vi "Test - Draw Teapot.vi"() -> ()   [LabVIEW 2022 SP3, in "Raster.lvlib"] (continued)
"v"=0.0}, "Colour"=12517256}, "Vertex 3"={"Position"={"x"=400.0, "y"=464.85934, "z"=0.98939073}, "UV"={"u"=0.0, "v"=0.0}, "Colour"=12517256}, "Alpha"=0.0, "Alpha Blending Enabled"=FALSE, "Colour"=12385414}, {"Vertex 1"={"Position"={"x"=261.91296, "y"=120.87895, "z"=0.98915625}, "UV"={"u"=0.0, "v"=0.0}, "Colour"=12517256}, "Vertex 2"={"Position"={"x"=278.23944, "y"=120.85737, "z"=0.98926175}, "UV"={"u"=0.0, "v"=0.0}, "Colour"=12517256}, "Vertex 3"={"Position"={"x"=278.11005, "y"=127.45417, "z"=0.9896591}, "UV"={"u"=0.0, "v"=0.0}, "Colour"=12517256}, "Alpha"=0.0, "Alpha Blending Enabled"=FALSE, "Colour"=131841}, {"Vertex 1"={"Position"={"x"=411.51666, "y"=449.75494, "z"=0.98939085}, "UV"={"u"=0.0, "v"=0.0}, "Colour"=12517256}, "Vertex 2"={"Position"={"x"=412.7883, "y"=456.74655, "z"=0.98931825}, "UV"={"u"=0.0, "v"=0.0}, "Colour"=12517256}, "Vertex 3"={"Position"={"x"=418.46112, "y"=456.03012, "z"=0.9893673}, "UV"={"u"=0.0, "v"=0.0}, "Colour"=12517256}, "Alpha"=0.0, "Alpha Blending Enabled"=FALSE, "Colour"=2240024}, {"Vertex 1"={"Position"={"x"=561.44336, "y"=135.88576, "z"=0.9895325}, "UV"={"u"=0.0, "v"=0.0}, "Colour"=12517256}, "Vertex 2"={"Position"={"x"=559.66595, "y"=133.57411, "z"=0.9895382}, "UV"={"u"=0.0, "v"=0.0}, "Colour"=12517256}, "Vertex 3"={"Position"={"x"=561.4089, "y"=125.13941, "z"=0.98900545}, "UV"={"u"=0.0, "v"=0.0}, "Colour"=12517256}, "Alpha"=0.0, "Alpha Blending Enabled"=FALSE, "Colour"=131841}, {"Vertex 1"={"Position"={"x"=358.07327, "y"=408.73547, "z"=0.9892421}, "UV"={"u"=0.0, "v"=0.0}, "Colour"=12517256}, "Vertex 2"={"Position"={"x"=369.4374, "y"=409.63797, "z"=0.98946077}, "UV"={"u"=0.0, "v"=0.0}, "Colour"=12517256}, "Vertex 3"={"Position"={"x"=374.2221, "y"=410.54718, "z"=0.98937297}, "UV"={"u"=0.0, "v"=0.0}, "Colour"=12517256}, "Alpha"=0.0, "Alpha Blending Enabled"=FALSE, "Colour"=10014061}, {"Vertex 1"={"Position"={"x"=238.15663, "y"=384.24957, "z"=0.9895312}, "UV"={"u"=0.0, "v"=0.0}, "Colour"=12517256}, "Vertex 2"={"Position"={"x"=240.3879, "y"=388.06317, "z"=0.98953843}, "UV"={"u"=0.0, "v"=0.0}, "Colour"=12517256}, "Vertex 3"={"Position"={"x"=238.64832, "y"=392.52478, "z"=0.9890058}, "UV"={"u"=0.0, "v"=0.0}, "Colour"=12517256}, "Alpha"=0.0, "Alpha Blending Enabled"=FALSE, "Colour"=6126658}, {"Vertex 1"={"Position"={"x"=414.14594, "y"=412.64026, "z"=0.98952574}, "UV"={"u"=0.0, "v"=0.0}, "Colour"=12517256}, "Vertex 2"={"Position"={"x"=420.22992, "y"=411.29608, "z"=0.9893006}, "UV"={"u"=0.0, "v"=0.0}, "Colour"=12517256}, "Vertex 3"={"Position"={"x"=414.01163, "y"=411.85974, "z"=0.9892462}, "UV"={"u"=0.0, "v"=0.0}, "Colour"=12517256}, "Alpha"=0.0, "Alpha Blending Enabled"=FALSE, "Colour"=10804598}, {"Vertex 1"={"Position"={"x"=412.7883, "y"=456.74655, "z"=0.98931825}, "UV"={"u"=0.0, "v"=0.0}, "Colour"=12517256}, "Vertex 2"={"Position"={"x"=411.51666, "y"=449.75494, "z"=0.98939085}, "UV"={"u"=0.0, "v"=0.0}, "Colour"=12517256}, "Vertex 3"={"Position"={"x"=405.94202, "y"=450.1419, "z"=0.98936325}, "UV"={"u"=0.0, "v"=0.0}, "Colour"=12517256}, "Alpha"=0.0, "Alpha Blending Enabled"=FALSE, "Colour"=2635293}, {"Vertex 1"={"Position"={"x"=400.0, "y"=462.5336, "z"=0.98927724}, "UV"={"u"=0.0, "v"=0.0}, "Colour"=12517256}, "Vertex 2"={"Position"={"x"=400.0, "y"=464.85934, "z"=0.98939073}, "UV"={"u"=0.0, "v"=0.0}, "Colour"=12517256}, "Vertex 3"={"Position"={"x"=405.62814, "y"=464.7204, "z"=0.9893997}, "UV"={"u"=0.0, "v"=0.0}, "Colour"=12517256}, "Alpha"=0.0, "Alpha Blending Enabled"=FALSE, "Colour"=12385414}, {"Vertex 1"={"Position"={"x"=240.33403, "y"=133.57411, "z"=0.9895382}, "UV"={"u"=0.0, "v"=0.0}, "Colour"=12517256}, "Vertex 2"={"Position"={"x"=238.55664, "y"=135.88576, "z"=0.9895325}, "UV"={"u"=0.0, "v"=0.0}, "Colour"=12517256}, "Vertex 3"={"Position"={"x"=236.70218, "y"=127.47084, "z"=0.9889933}, "UV"={"u"=0.0, "v"=0.0}, "Colour"=12517256}, "Alpha"=0.0, "Alpha Blending Enabled"=FALSE, "Colour"=131841}, {"Vertex 1"={"Position"={"x"=327.3322, "y"=123.64719, "z"=0.9895792}, "UV"={"u"=0.0, "v"=0.0}, "Colour"=12517256}, "Vertex 2"={"Position"={"x"=299.91116, "y"=121.74838, "z"=0.98940194}, "UV"={"u"=0.0, "v"=0.0}, "Colour"=12517256}, "Vertex 3"={"Position"={"x"=303.40628, "y"=116.389046, "z"=0.98908174}, "UV"={"u"=0.0, "v"=0.0}, "Colour"=12517256}, "Alpha"=0.0, "Alpha Blending Enabled"=FALSE, "Colour"=131841}, {"Vertex 1"={"Position"={"x"=559.61206, "y"=388.06317, "z"=0.98953843}, "UV"={"u"=0.0, "v"=0.0}, "Colour"=12517256}, "Vertex 2"={"Position"={"x"=561.8434, "y"=384.24957, "z"=0.9895312}, "UV"={"u"=0.0, "v"=0.0}, "Colour"=12517256}, "Vertex 3"={"Position"={"x"=563.7232, "y"=388.5807, "z"=0.9889904}, "UV"={"u"=0.0, "v"=0.0}, "Colour"=12517256}, "Alpha"=0.0, "Alpha Blending Enabled"=FALSE, "Colour"=6126658}, {"Vertex 1"={"Position"={"x"=561.8434, "y"=138.31693, "z"=0.9895312}, "UV"={"u"=0.0, "v"=0.0}, "Colour"=12517256}, "Vertex 2"={"Position"={"x"=561.44336, "y"=135.88576, "z"=0.9895325}, "UV"={"u"=0.0, "v"=0.0}, "Colour"=12517256}, "Vertex 3"={"Position"={"x"=563.29785, "y"=127.47084, "z"=0.9889933}, "UV"={"u"=0.0, "v"=0.0}, "Colour"=12517256}, "Alpha"=0.0, "Alpha Blending Enabled"=FALSE, "Colour"=658951}, {"Vertex 1"={"Position"={"x"=434.23392, "y"=122.73771, "z"=0.98956543}, "UV"={"u"=0.0, "v"=0.0}, "Colour"=12517256}, "Vertex 2"={"Position"={"x"=464.53143, "y"=116.20814, "z"=0.98913753}, "UV"={"u"=0.0, "v"=0.0}, "Colour"=12517256}, "Vertex 3"={"Position"={"x"=469.5572, "y"=119.82906, "z"=0.98935246}, "UV"={"u"=0.0, "v"=0.0}, "Colour"=12517256}, "Alpha"=0.0, "Alpha Blending Enabled"=FALSE, "Colour"=131841}, {"Vertex 1"={"Position"={"x"=238.55664, "y"=135.88576, "z"=0.9895325}, "UV"={"u"=0.0, "v"=0.0}, "Colour"=12517256}, "Vertex 2"={"Position"={"x"=238.15663, "y"=138.31693, "z"=0.9895312}, "UV"={"u"=0.0, "v"=0.0}, "Colour"=12517256}, "Vertex 3"={"Position"={"x"=236.27676, "y"=130.00505, "z"=0.9889904}, "UV"={"u"=0.0, "v"=0.0}, "Colour"=12517256}, "Alpha"=0.0, "Alpha Blending Enabled"=FALSE, "Colour"=658951}, {"Vertex 1"={"Position"={"x"=381.53885, "y"=456.03012, "z"=0.9893673}, "UV"={"u"=0.0, "v"=0.0}, "Colour"=12517256}, "Vertex 2"={"Position"={"x"=381.54898, "y"=461.16928, "z"=0.9893677}, "UV"={"u"=0.0, "v"=0.0}, "Colour"=12517256}, "Vertex 3"={"Position"={"x"=387.21857, "y"=461.90887, "z"=0.9893186}, "UV"={"u"=0.0, "v"=0.0}, "Colour"=12517256}, "Alpha"=0.0, "Alpha Blending Enabled"=FALSE, "Colour"=8234841}, {"Vertex 1"={"Position"={"x"=418.45102, "y"=461.16928, "z"=0.9893677}, "UV"={"u"=0.0, "v"=0.0}, "Colour"=12517256}, "Vertex 2"={"Position"={"x"=418.46112, "y"=456.03012, "z"=0.9893673}, "UV"={"u"=0.0, "v"=0.0}, "Colour"=12517256}, "Vertex 3"={"Position"={"x"=412.7883, "y"=456.74655, "z"=0.98931825}, "UV"={"u"=0.0, "v"=0.0}, "Colour"=12517256}, "Alpha"=0.0, "Alpha Blending Enabled"=FALSE, "Colour"=8234841}, {"Vertex 1"={"Position"={"x"=563.43286, "y"=141.19958, "z"=0.98952615}, "UV"={"u"=0.0, "v"=0.0}, "Colour"=12517256}, "Vertex 2"={"Position"={"x"=561.8434, "y"=138.31693, "z"=0.9895312}, "UV"={"u"=0.0, "v"=0.0}, "Colour"=12517256}, "Vertex 3"={"Position"={"x"=563.7232, "y"=130.00505, "z"=0.9889904}, "UV"={"u"=0.0, "v"=0.0}, "Colour"=12517256}, "Alpha"=0.0, "Alpha Blending Enabled"=FALSE, "Colour"=131841}, {"Vertex 1"={"Position"={"x"=393.39984, "y"=457.19626, "z"=0.9892875}, "UV"={"u"=0.0, "v"=0.0}, "Colour"=12517256}, "Vertex 2"={"Position"={"x"=394.058, "y"=450.1419, "z"=0.98936325}, "UV"={"u"=0.0, "v"=0.0}, "Colour"=12517256}, "Vertex 3"={"Position"={"x"=388.48337, "y"=449.75494, "z"=0.98939085}, "UV"={"u"=0.0, "v"=0.0}, "Colour"=12517256}, "Alpha"=0.0, "Alpha Blending Enabled"=FALSE, "Colour"=2635293}, {"Vertex 1"={"Position"={"x"=689.1351, "y"=288.03708, "z"=0.9894408}, "UV"={"u"=0.0, "v"=0.0}, "Colour"=12517256}, "Vertex 2"={"Position"={"x"=683.1556, "y"=265.8486, "z"=0.9893541}, "UV"={"u"=0.0, "v"=0.0}, "Colour"=12517256}, "Vertex 3"={"Position"={"x"=681.67114, "y"=272.51385, "z"=0.9892468}, "UV"={"u"=0.0, "v"=0.0}, "Colour"=12517256}, "Alpha"=0.0, "Alpha Blending Enabled"=FALSE, "Colour"=5336378}, {"Vertex 1"={"Position"={"x"=238.15663, "y"=138.31693, "z"=0.9895312}, "UV"={"u"=0.0, "v"=0.0}, "Colour"=12517256}, "Vertex 2"={"Position"={"x"=236.5671, "y"=141.19958, "z"=0.98952615}, "UV"={"u"=0.0, "v"=0.0}, "Colour"=12517256}, "Vertex 3"={"Position"={"x"=234.58522, "y"=132.95152, "z"=0.9889795}, "UV"={"u"=0.0, "v"=0.0}, "Colour"=12517256}, "Alpha"=0.0, "Alpha Blending Enabled"=FALSE, "Colour"=131841}, {"Vertex 1"={"Position"={"x"=390.2171, "y"=413.03857, "z"=0.9894885}, "UV"={"u"=0.0, "v"=0.0}, "Colour"=12517256}, "Vertex 2"={"Position"={"x"=385.98837, "y"=411.85974, "z"=0.9892462}, "UV"={"u"=0.0, "v"=0.0}, "Colour"=12517256}, "Vertex 3"={"Position"={"x"=379.77005, "y"=411.29608, "z"=0.9893006}, "UV"={"u"=0.0, "v"=0.0}, "Colour"=12517256}, "Alpha"=0.0, "Alpha Blending Enabled"=FALSE, "Colour"=10804598}, {"Vertex 1"={"Position"={"x"=681.67114, "y"=272.51385, "z"=0.9892468}, "UV"={"u"=0.0, "v"=0.0}, "Colour"=12517256}, "Vertex 2"={"Position"={"x"=687.13184, "y"=293.32037, "z"=0.9893478}, "UV"={"u"=0.0, "v"=0.0}, "Colour"=12517256}, "Vertex 3"={"Position"={"x"=689.1351, "y"=288.03708, "z"=0.9894408}, "UV"={"u"=0.0, "v"=0.0}, "Colour"=12517256}, "Alpha"=0.0, "Alpha Blending Enabled"=FALSE, "Colour"=5929280}, {"Vertex 1"={"Position"={"x"=410.90912, "y"=464.3185, "z"=0.98942566}, "UV"={"u"=0.0, "v"=0.0}, "Colour"=12517256}, "Vertex 2"={"Position"={"x"=412.78143, "y"=461.90887, "z"=0.9893186}, "UV"={"u"=0.0, "v"=0.0}, "Colour"=12517256}, "Vertex 3"={"Position"={"x"=406.59674, "y"=462.37308, "z"=0.9892879}, "UV"={"u"=0.0, "v"=0.0}, "Colour"=12517256}, "Alpha"=0.0, "Alpha Blending Enabled"=FALSE, "Colour"=12253573}, {"Vertex 1"={"Position"={"x"=521.76056, "y"=120.85737, "z"=0.98926175}, "UV"={"u"=0.0, "v"=0.0}, "Colour"=12517256}, "Vertex 2"={"Position"={"x"=538.08704, "y"=120.87895, "z"=0.98915625}, "UV"={"u"=0.0, "v"=0.0}, "Colour"=12517256}, "Vertex 3"={"Position"={"x"=537.5546, "y"=128.3227, "z"=0.989609}, "UV"={"u"=0.0, "v"=0.0}, "Colour"=12517256}, "Alpha"=0.0, "Alpha Blending Enabled"=FALSE, "Colour"=131841}, {"Vertex 1"={"Position"={"x"=229.65198, "y"=367.2159, "z"=0.9895041}, "UV"={"u"=0.0, "v"=0.0}, "Colour"=12517256}, "Vertex 2"={"Position"={"x"=238.15663, "y"=384.24957, "z"=0.9895312}, "UV"={"u"=0.0, "v"=0.0}, "Colour"=12517256}, "Vertex 3"={"Position"={"x"=236.27676, "y"=388.5807, "z"=0.9889904}, "UV"={"u"=0.0, "v"=0.0}, "Colour"=12517256}, "Alpha"=0.0, "Alpha Blending Enabled"=FALSE, "Colour"=5665598}, {"Vertex 1"={"Position"={"x"=567.755, "y"=144.99042, "z"=0.9895123}, "UV"={"u"=0.0, "v"=0.0}, "Colour"=12517256}, "Vertex 2"={"Position"={"x"=563.43286, "y"=141.19958, "z"=0.98952615}, "UV"={"u"=0.0, "v"=0.0}, "Colour"=12517256}, "Vertex 3"={"Position"={"x"=565.4148, "y"=132.95152, "z"=0.9889795}, "UV"={"u"=0.0, "v"=0.0}, "Colour"=12517256}, "Alpha"=0.0, "Alpha Blending Enabled"=FALSE, "Colour"=131841}, {"Vertex 1"={"Position"={"x"=536.943, "y"=391.80936, "z"=0.98916364}, "UV"={"u"=0.0, "v"=0.0}, "Colour"=12517256}, "Vertex 2"={"Position"={"x"=528.8192, "y"=395.14902, "z"=0.98921615}, "UV"={"u"=0.0, "v"=0.0}, "Colour"=12517256}, "Vertex 3"={"Position"={"x"=528.68146, "y"=391.44998, "z"=0.9896373}, "UV"={"u"=0.0, "v"=0.0}, "Colour"=12517256}, "Alpha"=0.0, "Alpha Blending Enabled"=FALSE, "Colour"=8893792}, {"Vertex 1"={"Position"={"x"=303.40628, "y"=116.389046, "z"=0.98908174}, "UV"={"u"=0.0, "v"=0.0}, "Colour"=12517256}, "Vertex 2"={"Position"={"x"=330.4428, "y"=119.82906, "z"=0.98935246}, "UV"={"u"=0.0, "v"=0.0}, "Colour"=12517256}, "Vertex 3"={"Position"={"x"=327.3322, "y"=123.64719, "z"=0.9895792}, "UV"={"u"=0.0, "v"=0.0}, "Colour"=12517256}, "Alpha"=0.0, "Alpha Blending Enabled"=FALSE, "Colour"=131841}, {"Vertex 1"={"Position"={"x"=615.98, "y"=270.86078, "z"=0.989385}, "UV"={"u"=0.0, "v"=0.0}, "Colour"=12517256}, "Vertex 2"={"Position"={"x"=635.5962, "y"=277.87793, "z"=0.989419}, "UV"={"u"=0.0, "v"=0.0}, "Colour"=12517256}, "Vertex 3"={"Position"={"x"=642.9325, "y"=269.1037, "z"=0.9892055}, "UV"={"u"=0.0, "v"=0.0}, "Colour"=12517256}, "Alpha"=0.0, "Alpha Blending Enabled"=FALSE, "Colour"=12253573}, {"Vertex 1"={"Position"={"x"=394.37186, "y"=464.7204, "z"=0.9893997}, "UV"={"u"=0.0, "v"=0.0}, "Colour"=12517256}, "Vertex 2"={"Position"={"x"=393.40326, "y"=462.37308, "z"=0.9892879}, "UV"={"u"=0.0, "v"=0.0}, "Colour"=12517256}, "Vertex 3"={"Position"={"x"=387.21857, "y"=461.90887, "z"=0.9893186}, "UV"={"u"=0.0, "v"=0.0}, "Colour"=12517256}, "Alpha"=0.0, "Alpha Blending Enabled"=FALSE, "Colour"=12253573}, {"Vertex 1"={"Position"={"x"=406.60013, "y"=457.19626, "z"=0.9892875}, "UV"={"u"=0.0, "v"=0.0}, "Colour"=12517256}, "Vertex 2"={"Position"={"x"=405.94202, "y"=450.1419, "z"=0.98936325}, "UV"={"u"=0.0, "v"=0.0}, "Colour"=12517256}, "Vertex 3"={"Position"={"x"=400.0, "y"=450.27567, "z"=0.9893538}, "UV"={"u"=0.0, "v"=0.0}, "Colour"=12517256}, "Alpha"=0.0, "Alpha Blending Enabled"=FALSE, "Colour"=2832671}, {"Vertex 1"={"Position"={"x"=412.7883, "y"=456.74655, "z"=0.98931825}, "UV"={"u"=0.0, "v"=0.0}, "Colour"=12517256}, "Vertex 2"={"Position"={"x"=412.78143, "y"=461.90887, "z"=0.9893186}, "UV"={"u"=0.0, "v"=0.0}, "Colour"=12517256}, "Vertex 3"={"Position"={"x"=418.45102, "y"=461.16928, "z"=0.9893677}, "UV"={"u"=0.0, "v"=0.0}, "Colour"=12517256}, "Alpha"=0.0, "Alpha Blending Enabled"=FALSE, "Colour"=8234841}, {"Vertex 1"={"Position"={"x"=387.21857, "y"=461.90887, "z"=0.9893186}, "UV"={"u"=0.0, "v"=0.0}, "Colour"=12517256}, "Vertex 2"={"Position"={"x"=387.2117, "y"=456.74655, "z"=0.98931825}, "UV"={"u"=0.0, "v"=0.0}, "Colour"=12517256}, "Vertex 3"={"Position"={"x"=381.53885, "y"=456.03012, "z"=0.9893673}, "UV"={"u"=0.0, "v"=0.0}, "Colour"=12517256}, "Alpha"=0.0, "Alpha Blending Enabled"=FALSE, "Colour"=8234841}, {"Vertex 1"={"Position"={"x"=388.48337, "y"=449.75494, "z"=0.98939085}, "UV"={"u"=0.0, "v"=0.0}, "Colour"=12517256}, "Vertex 2"={"Position"={"x"=387.2117, "y"=456.74655, "z"=0.98931825}, "UV"={"u"=0.0, "v"=0.0}, "Colour"=12517256}, "Vertex 3"={"Position"={"x"=393.39984, "y"=457.19626, "z"=0.9892875}, "UV"={"u"=0.0, "v"=0.0}, "Colour"=12517256}, "Alpha"=0.0, "Alpha Blending Enabled"=FALSE, "Colour"=2635293}, {"Vertex 1"={"Position"={"x"=400.0, "y"=457.35184, "z"=0.9892768}, "UV"={"u"=0.0, "v"=0.0}, "Colour"=12517256}, "Vertex 2"={"Position"={"x"=400.0, "y"=450.27567, "z"=0.9893538}, "UV"={"u"=0.0, "v"=0.0}, "Colour"=12517256}, "Vertex 3"={"Position"={"x"=394.058, "y"=450.1419, "z"=0.98936325}, "UV"={"u"=0.0, "v"=0.0}, "Colour"=12517256}, "Alpha"=0.0, "Alpha Blending Enabled"=FALSE, "Colour"=2832671}, {"Vertex 1"={"Position"={"x"=271.1808, "y"=395.14902, "z"=0.98921615}, "UV"={"u"=0.0, "v"=0.0}, "Colour"=12517256}, "Vertex 2"={"Position"={"x"=263.057, "y"=391.80936, "z"=0.98916364}, "UV"={"u"=0.0, "v"=0.0}, "Colour"=12517256}, "Vertex 3"={"Position"={"x"=263.53796, "y"=388.02435, "z"=0.98961246}, "UV"={"u"=0.0, "v"=0.0}, "Colour"=12517256}, "Alpha"=0.0, "Alpha Blending Enabled"=FALSE, "Colour"=8893792}, {"Vertex 1"={"Position"={"x"=236.5671, "y"=141.19958, "z"=0.98952615}, "UV"={"u"=0.0, "v"=0.0}, "Colour"=12517256}, "Vertex 2"={"Position"={"x"=232.24501, "y"=144.99042, "z"=0.9895123}, "UV"={"u"=0.0, "v"=0.0}, "Colour"=12517256}, "Vertex 3"={"Position"={"x"=229.97716, "y"=136.71501, "z"=0.9889498}, "UV"={"u"=0.0, "v"=0.0}, "Colour"=12517256}, "Alpha"=0.0, "Alpha Blending Enabled"=FALSE, "Colour"=131841}, {"Vertex 1"={"Position"={"x"=342.35834, "y"=112.87481, "z"=0.9889396}, "UV"={"u"=0.0, "v"=0.0}, "Colour"=12517256}, "Vertex 2"={"Position"={"x"=369.6793, "y"=121.04659, "z"=0.9894655}, "UV"={"u"=0.0, "v"=0.0}, "Colour"=12517256}, "Vertex 3"={"Position"={"x"=365.76608, "y"=122.73771, "z"=0.98956543}, "UV"={"u"=0.0, "v"=0.0}, "Colour"=12517256}, "Alpha"=0.0, "Alpha Blending Enabled"=FALSE, "Colour"=131841}, {"Vertex 1"={"Position"={"x"=405.94202, "y"=450.1419, "z"=0.98936325}, "UV"={"u"=0.0, "v"=0.0}, "Colour"=12517256}, "Vertex 2"={"Position"={"x"=406.60013, "y"=457.19626, "z"=0.9892875}, "UV"={"u"=0.0, "v"=0.0}, "Colour"=12517256}, "Vertex 3"={"Position"={"x"=412.7883, "y"=456.74655, "z"=0.98931825}, "UV"={"u"=0.0, "v"=0.0}, "Colour"=12517256}, "Alpha"=0.0, "Alpha Blending Enabled"=FALSE, "Colour"=2635293}, {"Vertex 1"={"Position"={"x"=561.8434, "y"=384.24957, "z"=0.9895312}, "UV"={"u"=0.0, "v"=0.0}, "Colour"=12517256}, "Vertex 2"={"Position"={"x"=570.348, "y"=367.2159, "z"=0.9895041}, "UV"={"u"=0.0, "v"=0.0}, "Colour"=12517256}, "Vertex 3"={"Position"={"x"=572.7935, "y"=370.8628, "z"=0.98893183}, "UV"={"u"=0.0, "v"=0.0}, "Colour"=12517256}, "Alpha"=0.0, "Alpha Blending Enabled"=FALSE, "Colour"=5665598}, {"Vertex 1"={"Position"={"x"=405.62814, "y"=464.7204, "z"=0.9893997}, "UV"={"u"=0.0, "v"=0.0}, "Colour"=12517256}, "Vertex 2"={"Position"={"x"=406.59674, "y"=462.37308, "z"=0.9892879}, "UV"={"u"=0.0, "v"=0.0}, "Colour"=12517256}, "Vertex 3"={"Position"={"x"=400.0, "y"=462.5336, "z"=0.98927724}, "UV"={"u"=0.0, "v"=0.0}, "Colour"=12517256}, "Alpha"=0.0, "Alpha Blending Enabled"=FALSE, "Colour"=12385414}, {"Vertex 1"={"Position"={"x"=653.6545, "y"=220.1329, "z"=0.989419}, "UV"={"u"=0.0, "v"=0.0}, "Colour"=12517256}, "Vertex 2"={"Position"={"x"=626.93384, "y"=205.09799, "z"=0.989385}, "UV"={"u"=0.0, "v"=0.0}, "Colour"=12517256}, "Vertex 3"={"Position"={"x"=630.16, "y"=212.58409, "z"=0.9891591}, "UV"={"u"=0.0, "v"=0.0}, "Colour"=12517256}, "Alpha"=0.0, "Alpha Blending Enabled"=FALSE, "Colour"=131841}, {"Vertex 1"={"Position"={"x"=400.0, "y"=464.85934, "z"=0.98939073}, "UV"={"u"=0.0, "v"=0.0}, "Colour"=12517256}, "Vertex 2"={"Position"={"x"=400.0, "y"=462.5336, "z"=0.98927724}, "UV"={"u"=0.0, "v"=0.0}, "Colour"=12517256}, "Vertex 3"={"Position"={"x"=393.40326, "y"=462.37308, "z"=0.9892879}, "UV"={"u"=0.0, "v"=0.0}, "Colour"=12517256}, "Alpha"=0.0, "Alpha Blending Enabled"=FALSE, "Colour"=12385414}, {"Vertex 1"={"Position"={"x"=574.1452, "y"=149.78308, "z"=0.9894918}, "UV"={"u"=0.0, "v"=0.0}, "Colour"=12517256}, "Vertex 2"={"Position"={"x"=567.755, "y"=144.99042, "z"=0.9895123}, "UV"={"u"=0.0, "v"=0.0}, "Colour"=12517256}, "Vertex 3"={"Position"={"x"=570.0229, "y"=136.71501, "z"=0.9889498}, "UV"={"u"=0.0, "v"=0.0}, "Colour"=12517256}, "Alpha"=0.0, "Alpha Blending Enabled"=FALSE, "Colour"=131841}, {"Vertex 1"={"Position"={"x"=435.4722, "y"=409.9763, "z"=0.9891187}, "UV"={"u"=0.0, "v"=0.0}, "Colour"=12517256}, "Vertex 2"={"Position"={"x"=425.77792, "y"=410.54718, "z"=0.98937297}, "UV"={"u"=0.0, "v"=0.0}, "Colour"=12517256}, "Vertex 3"={"Position"={"x"=430.5626, "y"=409.63797, "z"=0.98946077}, "UV"={"u"=0.0, "v"=0.0}, "Colour"=12517256}, "Alpha"=0.0, "Alpha Blending Enabled"=FALSE, "Colour"=10014061}, {"Vertex 1"={"Position"={"x"=677.2564, "y"=305.0474, "z"=0.9893478}, "UV"={"u"=0.0, "v"=0.0}, "Colour"=12517256}, "Vertex 2"={"Position"={"x"=672.2607, "y"=287.7658, "z"=0.9892468}, "UV"={"u"=0.0, "v"=0.0}, "Colour"=12517256}, "Vertex 3"={"Position"={"x"=665.27704, "y"=294.82538, "z"=0.9893541}, "UV"={"u"=0.0, "v"=0.0}, "Colour"=12517256}, "Alpha"=0.0, "Alpha Blending Enabled"=FALSE, "Colour"=11001719}, {"Vertex 1"={"Position"={"x"=656.14374, "y"=226.85892, "z"=0.9892055}, "UV"={"u"=0.0, "v"=0.0}, "Colour"=12517256}, "Vertex 2"={"Position"={"x"=672.9877, "y"=245.0455, "z"=0.9892731}, "UV"={"u"=0.0, "v"=0.0}, "Colour"=12517256}, "Vertex 3"={"Position"={"x"=671.18396, "y"=239.12437, "z"=0.9894685}, "UV"={"u"=0.0, "v"=0.0}, "Colour"=12517256}, "Alpha"=0.0, "Alpha Blending Enabled"=FALSE, "Colour"=592646}, {"Vertex 1"={"Position"={"x"=409.7829, "y"=413.03857, "z"=0.9894885}, "UV"={"u"=0.0, "v"=0.0}, "Colour"=12517256}, "Vertex 2"={"Position"={"x"=414.01163, "y"=411.85974, "z"=0.9892462}, "UV"={"u"=0.0, "v"=0.0}, "Colour"=12517256}, "Vertex 3"={"Position"={"x"=407.2289, "y"=412.21408, "z"=0.989212}, "UV"={"u"=0.0, "v"=0.0}, "Colour"=12517256}, "Alpha"=0.0, "Alpha Blending Enabled"=FALSE, "Colour"=10936183}, {"Vertex 1"={"Position"={"x"=352.83286, "y"=407.3197, "z"=0.98938274}, "UV"={"u"=0.0, "v"=0.0}, "Colour"=12517256}, "Vertex 2"={"Position"={"x"=338.4212, "y"=406.58887, "z"=0.98917925}, "UV"={"u"=0.0, "v"=0.0}, "Colour"=12517256}, "Vertex 3"={"Position"={"x"=333.56543, "y"=404.58322, "z"=0.98938376}, "UV"={"u"=0.0, "v"=0.0}, "Colour"=12517256}, "Alpha"=0.0, "Alpha Blending Enabled"=FALSE, "Colour"=9486695}, {"Vertex 1"={"Position"={"x"=485.95386, "y"=401.00818, "z"=0.9894933}, "UV"={"u"=0.0, "v"=0.0}, "Colour"=12517256}, "Vertex 2"={"Position"={"x"=502.10248, "y"=399.48126, "z"=0.9893889}, "UV"={"u"=0.0, "v"=0.0}, "Colour"=12517256}, "Vertex 3"={"Position"={"x"=498.59668, "y"=402.53433, "z"=0.9890617}, "UV"={"u"=0.0, "v"=0.0}, "Colour"=12517256}, "Alpha"=0.0, "Alpha Blending Enabled"=FALSE, "Colour"=9289061}, {"Vertex 1"={"Position"={"x"=394.058, "y"=450.1419, "z"=0.98936325}, "UV"={"u"=0.0, "v"=0.0}, "Colour"=12517256}, "Vertex 2"={"Position"={"x"=393.39984, "y"=457.19626, "z"=0.9892875}, "UV"={"u"=0.0, "v"=0.0}, "Colour"=12517256}, "Vertex 3"={"Position"={"x"=400.0, "y"=457.35184, "z"=0.9892768}, "UV"={"u"=0.0, "v"=0.0}, "Colour"=12517256}, "Alpha"=0.0, "Alpha Blending Enabled"=FALSE, "Colour"=2832671}, {"Vertex 1"={"Position"={"x"=387.2117, "y"=456.74655, "z"=0.98931825}, "UV"={"u"=0.0, "v"=0.0}, "Colour"=12517256}, "Vertex 2"={"Position"={"x"=387.21857, "y"=461.90887, "z"=0.9893186}, "UV"={"u"=0.0, "v"=0.0}, "Colour"=12517256}, "Vertex 3"={"Position"={"x"=393.40326, "y"=462.37308, "z"=0.9892879}, "UV"={"u"=0.0, "v"=0.0}, "Colour"=12517256}, "Alpha"=0.0, "Alpha Blending Enabled"=FALSE, "Colour"=8630366}, {"Vertex 1"={"Position"={"x"=412.78143, "y"=461.90887, "z"=0.9893186}, "UV"={"u"=0.0, "v"=0.0}, "Colour"=12517256}, "Vertex 2"={"Position"={"x"=412.7883, "y"=456.74655, "z"=0.98931825}, "UV"={"u"=0.0, "v"=0.0}, "Colour"=12517256}, "Vertex 3"={"Position"={"x"=406.60013, "y"=457.19626, "z"=0.9892875}, "UV"={"u"=0.0, "v"=0.0}, "Colour"=12517256}, "Alpha"=0.0, "Alpha Blending Enabled"=FALSE, "Colour"=8630366}, {"Vertex 1"={"Position"={"x"=394.9576, "y"=413.28833, "z"=0.9894651}, "UV"={"u"=0.0, "v"=0.0}, "Colour"=12517256}, "Vertex 2"={"Position"={"x"=392.7711, "y"=412.21408, "z"=0.989212}, "UV"={"u"=0.0, "v"=0.0}, "Colour"=12517256}, "Vertex 3"={"Position"={"x"=385.98837, "y"=411.85974, "z"=0.9892462}, "UV"={"u"=0.0, "v"=0.0}, "Colour"=12517256}, "Alpha"=0.0, "Alpha Blending Enabled"=FALSE, "Colour"=10936183}, {"Vertex 1"={"Position"={"x"=539.9189, "y"=387.34802, "z"=0.98914444}, "UV"={"u"=0.0, "v"=0.0}, "Colour"=12517256}, "Vertex 2"={"Position"={"x"=536.943, "y"=391.80936, "z"=0.98916364}, "UV"={"u"=0.0, "v"=0.0}, "Colour"=12517256}, "Vertex 3"={"Position"={"x"=536.46204, "y"=388.02435, "z"=0.98961246}, "UV"={"u"=0.0, "v"=0.0}, "Colour"=12517256}, "Alpha"=0.0, "Alpha Blending Enabled"=FALSE, "Colour"=6456134}, {"Vertex 1"={"Position"={"x"=400.0, "y"=450.27567, "z"=0.9893538}, "UV"={"u"=0.0, "v"=0.0}, "Colour"=12517256}, "Vertex 2"={"Position"={"x"=400.0, "y"=457.35184, "z"=0.9892768}, "UV"={"u"=0.0, "v"=0.0}, "Colour"=12517256}, "Vertex 3"={"Position"={"x"=406.60013, "y"=457.19626, "z"=0.9892875}, "UV"={"u"=0.0, "v"=0.0}, "Colour"=12517256}, "Alpha"=0.0, "Alpha Blending Enabled"=FALSE, "Colour"=2832671}, {"Vertex 1"={"Position"={"x"=588.6202, "y"=267.82214, "z"=0.9893725}, "UV"={"u"=0.0, "v"=0.0}, "Colour"=12517256}, "Vertex 2"={"Position"={"x"=615.98, "y"=270.86078, "z"=0.989385}, "UV"={"u"=0.0, "v"=0.0}, "Colour"=12517256}, "Vertex 3"={"Position"={"x"=622.13776, "y"=260.7466, "z"=0.9891591}, "UV"={"u"=0.0, "v"=0.0}, "Colour"=12517256}, "Alpha"=0.0, "Alpha Blending Enabled"=FALSE, "Colour"=12451463}, {"Vertex 1"={"Position"={"x"=221.27509, "y"=350.14075, "z"=0.9894772}, "UV"={"u"=0.0, "v"=0.0}, "Colour"=12517256}, "Vertex 2"={"Position"={"x"=229.65198, "y"=367.2159, "z"=0.9895041}, "UV"={"u"=0.0, "v"=0.0}, "Colour"=12517256}, "Vertex 3"={"Position"={"x"=227.20647, "y"=370.8628, "z"=0.98893183}, "UV"={"u"=0.0, "v"=0.0}, "Colour"=12517256}, "Alpha"=0.0, "Alpha Blending Enabled"=FALSE, "Colour"=5599805}, {"Vertex 1"={"Position"={"x"=263.057, "y"=391.80936, "z"=0.98916364}, "UV"={"u"=0.0, "v"=0.0}, "Colour"=12517256}, "Vertex 2"={"Position"={"x"=260.08112, "y"=387.34802, "z"=0.98914444}, "UV"={"u"=0.0, "v"=0.0}, "Colour"=12517256}, "Vertex 3"={"Position"={"x"=260.69736, "y"=383.67197, "z"=0.98960334}, "UV"={"u"=0.0, "v"=0.0}, "Colour"=12517256}, "Alpha"=0.0, "Alpha Blending Enabled"=FALSE, "Colour"=6456134}, {"Vertex 1"={"Position"={"x"=672.2607, "y"=287.7658, "z"=0.9892468}, "UV"={"u"=0.0, "v"=0.0}, "Colour"=12517256}, "Vertex 2"={"Position"={"x"=677.2564, "y"=305.0474, "z"=0.9893478}, "UV"={"u"=0.0, "v"=0.0}, "Colour"=12517256}, "Vertex 3"={"Position"={"x"=683.021, "y"=299.1815, "z"=0.98931646}, "UV"={"u"=0.0, "v"=0.0}, "Colour"=12517256}, "Alpha"=0.0, "Alpha Blending Enabled"=FALSE, "Colour"=10870390}, {"Vertex 1"={"Position"={"x"=232.24501, "y"=144.99042, "z"=0.9895123}, "UV"={"u"=0.0, "v"=0.0}, "Colour"=12517256}, "Vertex 2"={"Position"={"x"=225.85475, "y"=149.78308, "z"=0.9894918}, "UV"={"u"=0.0, "v"=0.0}, "Colour"=12517256}, "Vertex 3"={"Position"={"x"=223.14096, "y"=141.4411, "z"=0.98890555}, "UV"={"u"=0.0, "v"=0.0}, "Colour"=12517256}, "Alpha"=0.0, "Alpha Blending Enabled"=FALSE, "Colour"=131841}, {"Vertex 1"={"Position"={"x"=626.93384, "y"=205.09799, "z"=0.989385}, "UV"={"u"=0.0, "v"=0.0}, "Colour"=12517256}, "Vertex 2"={"Position"={"x"=588.6202, "y"=195.32538, "z"=0.9893725}, "UV"={"u"=0.0, "v"=0.0}, "Colour"=12517256}, "Vertex 3"={"Position"={"x"=592.6936, "y"=203.5383, "z"=0.98914194}, "UV"={"u"=0.0, "v"=0.0}, "Colour"=12517256}, "Alpha"=0.0, "Alpha Blending Enabled"=FALSE, "Colour"=131841}, {"Vertex 1"={"Position"={"x"=656.72955, "y"=280.77734, "z"=0.9892731}, "UV"={"u"=0.0, "v"=0.0}, "Colour"=12517256}, "Vertex 2"={"Position"={"x"=642.9325, "y"=269.1037, "z"=0.9892055}, "UV"={"u"=0.0, "v"=0.0}, "Colour"=12517256}, "Vertex 3"={"Position"={"x"=635.5962, "y"=277.87793, "z"=0.989419}, "UV"={"u"=0.0, "v"=0.0}, "Colour"=12517256}, "Alpha"=0.0, "Alpha Blending Enabled"=FALSE, "Colour"=11594878}, {"Vertex 1"={"Position"={"x"=406.60013, "y"=457.19626, "z"=0.9892875}, "UV"={"u"=0.0, "v"=0.0}, "Colour"=12517256}, "Vertex 2"={"Position"={"x"=406.59674, "y"=462.37308, "z"=0.9892879}, "UV"={"u"=0.0, "v"=0.0}, "Colour"=12517256}, "Vertex 3"={"Position"={"x"=412.78143, "y"=461.90887, "z"=0.9893186}, "UV"={"u"=0.0, "v"=0.0}, "Colour"=12517256}, "Alpha"=0.0, "Alpha Blending Enabled"=FALSE, "Colour"=8630366}, {"Vertex 1"={"Position"={"x"=393.40326, "y"=462.37308, "z"=0.9892879}, "UV"={"u"=0.0, "v"=0.0}, "Colour"=12517256}, "Vertex 2"={"Position"={"x"=393.39984, "y"=457.19626, "z"=0.9892875}, "UV"={"u"=0.0, "v"=0.0}, "Colour"=12517256}, "Vertex 3"={"Position"={"x"=387.2117, "y"=456.74655, "z"=0.98931825}, "UV"={"u"=0.0, "v"=0.0}, "Colour"=12517256}, "Alpha"=0.0, "Alpha Blending Enabled"=FALSE, "Colour"=8630366}, {"Vertex 1"={"Position"={"x"=405.04242, "y"=413.28833, "z"=0.9894651}, "UV"={"u"=0.0, "v"=0.0}, "Colour"=12517256}, "Vertex 2"={"Position"={"x"=407.2289, "y"=412.21408, "z"=0.989212}, "UV"={"u"=0.0, "v"=0.0}, "Colour"=12517256}, "Vertex 3"={"Position"={"x"=400.0, "y"=412.3368, "z"=0.9892001}, "UV"={"u"=0.0, "v"=0.0}, "Colour"=12517256}, "Alpha"=0.0, "Alpha Blending Enabled"=FALSE, "Colour"=11002232}, {"Vertex 1"={"Position"={"x"=677.8947, "y"=280.0732, "z"=0.9892106}, "UV"={"u"=0.0, "v"=0.0}, "Colour"=12517256}, "Vertex 2"={"Position"={"x"=683.021, "y"=299.1815, "z"=0.98931646}, "UV"={"u"=0.0, "v"=0.0}, "Colour"=12517256}, "Vertex 3"={"Position"={"x"=687.13184, "y"=293.32037, "z"=0.9893478}, "UV"={"u"=0.0, "v"=0.0}, "Colour"=12517256}, "Alpha"=0.0, "Alpha Blending Enabled"=FALSE, "Colour"=8893793}, {"Vertex 1"={"Position"={"x"=656.72955, "y"=280.77734, "z"=0.9892731}, "UV"={"u"=0.0, "v"=0.0}, "Colour"=12517256}, "Vertex 2"={"Position"={"x"=665.27704, "y"=294.82538, "z"=0.9893541}, "UV"={"u"=0.0, "v"=0.0}, "Colour"=12517256}, "Vertex 3"={"Position"={"x"=672.2607, "y"=287.7658, "z"=0.9892468}, "UV"={"u"=0.0, "v"=0.0}, "Colour"=12517256}, "Alpha"=0.0, "Alpha Blending Enabled"=FALSE, "Colour"=11463293}, {"Vertex 1"={"Position"={"x"=400.0, "y"=413.3747, "z"=0.9894571}, "UV"={"u"=0.0, "v"=0.0}, "Colour"=12517256}, "Vertex 2"={"Position"={"x"=400.0, "y"=412.3368, "z"=0.9892001}, "UV"={"u"=0.0, "v"=0.0}, "Colour"=12517256}, "Vertex 3"={"Position"={"x"=392.7711, "y"=412.21408, "z"=0.989212}, "UV"={"u"=0.0, "v"=0.0}, "Colour"=12517256}, "Alpha"=0.0, "Alpha Blending Enabled"=FALSE, "Colour"=11002232}, {"Vertex 1"={"Position"={"x"=581.9382, "y"=155.67198, "z"=0.9894669}, "UV"={"u"=0.0, "v"=0.0}, "Colour"=12517256}, "Vertex 2"={"Position"={"x"=574.1452, "y"=149.78308, "z"=0.9894918}, "UV"={"u"=0.0, "v"=0.0}, "Colour"=12517256}, "Vertex 3"={"Position"={"x"=576.8591, "y"=141.4411, "z"=0.98890555}, "UV"={"u"=0.0, "v"=0.0}, "Colour"=12517256}, "Alpha"=0.0, "Alpha Blending Enabled"=FALSE, "Colour"=131841}, {"Vertex 1"={"Position"={"x"=570.348, "y"=367.2159, "z"=0.9895041}, "UV"={"u"=0.0, "v"=0.0}, "Colour"=12517256}, "Vertex 2"={"Position"={"x"=578.7249, "y"=350.14075, "z"=0.9894772}, "UV"={"u"=0.0, "v"=0.0}, "Colour"=12517256}, "Vertex 3"={"Position"={"x"=581.77545, "y"=353.0026, "z"=0.9888737}, "UV"={"u"=0.0, "v"=0.0}, "Colour"=12517256}, "Alpha"=0.0, "Alpha Blending Enabled"=FALSE, "Colour"=5599805}, {"Vertex 1"={"Position"={"x"=393.39984, "y"=457.19626, "z"=0.9892875}, "UV"={"u"=0.0, "v"=0.0}, "Colour"=12517256}, "Vertex 2"={"Position"={"x"=393.40326, "y"=462.37308, "z"=0.9892879}, "UV"={"u"=0.0, "v"=0.0}, "Colour"=12517256}, "Vertex 3"={"Position"={"x"=400.0, "y"=462.5336, "z"=0.98927724}, "UV"={"u"=0.0, "v"=0.0}, "Colour"=12517256}, "Alpha"=0.0, "Alpha Blending Enabled"=FALSE, "Colour"=8893792}, {"Vertex 1"={"Position"={"x"=406.59674, "y"=462.37308, "z"=0.9892879}, "UV"={"u"=0.0, "v"=0.0}, "Colour"=12517256}, "Vertex 2"={"Position"={"x"=406.60013, "y"=457.19626, "z"=0.9892875}, "UV"={"u"=0.0, "v"=0.0}, "Colour"=12517256}, "Vertex 3"={"Position"={"x"=400.0, "y"=457.35184, "z"=0.9892768}, "UV"={"u"=0.0, "v"=0.0}, "Colour"=12517256}, "Alpha"=0.0, "Alpha Blending Enabled"=FALSE, "Colour"=8893792}, {"Vertex 1"={"Position"={"x"=250.35448, "y"=121.69325, "z"=0.9890815}, "UV"={"u"=0.0, "v"=0.0}, "Colour"=12517256}, "Vertex 2"={"Position"={"x"=261.91296, "y"=120.87895, "z"=0.98915625}, "UV"={"u"=0.0, "v"=0.0}, "Colour"=12517256}, "Vertex 3"={"Position"={"x"=262.44534, "y"=128.3227, "z"=0.989609}, "UV"={"u"=0.0, "v"=0.0}, "Colour"=12517256}, "Alpha"=0.0, "Alpha Blending Enabled"=FALSE, "Colour"=131841}, {"Vertex 1"={"Position"={"x"=400.0, "y"=457.35184, "z"=0.9892768}, "UV"={"u"=0.0, "v"=0.0}, "Colour"=12517256}, "Vertex 2"={"Position"={"x"=400.0, "y"=462.5336, "z"=0.98927724}, "UV"={"u"=0.0, "v"=0.0}, "Colour"=12517256}, "Vertex 3"={"Position"={"x"=406.59674, "y"=462.37308, "z"=0.9892879}, "UV"={"u"=0.0, "v"=0.0}, "Colour"=12517256}, "Alpha"=0.0, "Alpha Blending Enabled"=FALSE, "Colour"=8893792}, {"Vertex 1"={"Position"={"x"=400.0, "y"=462.5336, "z"=0.98927724}, "UV"={"u"=0.0, "v"=0.0}, "Colour"=12517256}, "Vertex 2"={"Position"={"x"=400.0, "y"=457.35184, "z"=0.9892768}, "UV"={"u"=0.0, "v"=0.0}, "Colour"=12517256}, "Vertex 3"={"Position"={"x"=393.39984, "y"=457.19626, "z"=0.9892875}, "UV"={"u"=0.0, "v"=0.0}, "Colour"=12517256}, "Alpha"=0.0, "Alpha Blending Enabled"=FALSE, "Colour"=8893792}, {"Vertex 1"={"Position"={"x"=469.5572, "y"=119.82906, "z"=0.98935246}, "UV"={"u"=0.0, "v"=0.0}, "Colour"=12517256}, "Vertex 2"={"Position"={"x"=496.59372, "y"=116.389046, "z"=0.98908174}, "UV"={"u"=0.0, "v"=0.0}, "Colour"=12517256}, "Vertex 3"={"Position"={"x"=500.08884, "y"=121.74838, "z"=0.98940194}, "UV"={"u"=0.0, "v"=0.0}, "Colour"=12517256}, "Alpha"=0.0, "Alpha Blending Enabled"=FALSE, "Colour"=131841}, {"Vertex 1"={"Position"={"x"=430.5626, "y"=409.63797, "z"=0.98946077}, "UV"={"u"=0.0, "v"=0.0}, "Colour"=12517256}, "Vertex 2"={"Position"={"x"=441.92676, "y"=408.73547, "z"=0.9892421}, "UV"={"u"=0.0, "v"=0.0}, "Colour"=12517256}, "Vertex 3"={"Position"={"x"=435.4722, "y"=409.9763, "z"=0.9891187}, "UV"={"u"=0.0, "v"=0.0}, "Colour"=12517256}, "Alpha"=0.0, "Alpha Blending Enabled"=FALSE, "Colour"=10014061}, {"Vertex 1"={"Position"={"x"=538.08704, "y"=120.87895, "z"=0.98915625}, "UV"={"u"=0.0, "v"=0.0}, "Colour"=12517256}, "Vertex 2"={"Position"={"x"=549.6455, "y"=121.69325, "z"=0.9890815}, "UV"={"u"=0.0, "v"=0.0}, "Colour"=12517256}, "Vertex 3"={"Position"={"x"=548.5519, "y"=129.69556, "z"=0.9895737}, "UV"={"u"=0.0, "v"=0.0}, "Colour"=12517256}, "Alpha"=0.0, "Alpha Blending Enabled"=FALSE, "Colour"=131841}, {"Vertex 1"={"Position"={"x"=225.85475, "y"=149.78308, "z"=0.9894918}, "UV"={"u"=0.0, "v"=0.0}, "Colour"=12517256}, "Vertex 2"={"Position"={"x"=218.06183, "y"=155.67198, "z"=0.9894669}, "UV"={"u"=0.0, "v"=0.0}, "Colour"=12517256}, "Vertex 3"={"Position"={"x"=214.76619, "y"=147.27748, "z"=0.9888514}, "UV"={"u"=0.0, "v"=0.0}, "Colour"=12517256}, "Alpha"=0.0, "Alpha Blending Enabled"=FALSE, "Colour"=131841}, {"Vertex 1"={"Position"={"x"=687.13184, "y"=293.32037, "z"=0.9893478}, "UV"={"u"=0.0, "v"=0.0}, "Colour"=12517256}, "Vertex 2"={"Position"={"x"=681.67114, "y"=272.51385, "z"=0.9892468}, "UV"={"u"=0.0, "v"=0.0}, "Colour"=12517256}, "Vertex 3"={"Position"={"x"=677.8947, "y"=280.0732, "z"=0.9892106}, "UV"={"u"=0.0, "v"=0.0}, "Colour"=12517256}, "Alpha"=0.0, "Alpha Blending Enabled"=FALSE, "Colour"=8498524}, {"Vertex 1"={"Position"={"x"=338.4212, "y"=406.58887, "z"=0.98917925}, "UV"={"u"=0.0, "v"=0.0}, "Colour"=12517256}, "Vertex 2"={"Position"={"x"=352.83286, "y"=407.3197, "z"=0.98938274}, "UV"={"u"=0.0, "v"=0.0}, "Colour"=12517256}, "Vertex 3"={"Position"={"x"=358.07327, "y"=408.73547, "z"=0.9892421}, "UV"={"u"=0.0, "v"=0.0}, "Colour"=12517256}, "Alpha"=0.0, "Alpha Blending Enabled"=FALSE, "Colour"=9684329}, {"Vertex 1"={"Position"={"x"=213.20128, "y"=333.07422, "z"=0.9894514}, "UV"={"u"=0.0, "v"=0.0}, "Colour"=12517256}, 
